vi "Run Multiple Bitfiles.vi"(8 "error in (no error)":errorcluster, 11 "rt data in":T1 {"Compiled Data"."FPGA Data"."1.1 APUs"."shared settings"."cycle start" format="%#.15g"; "Compiled Data"."FPGA Data"."1.0 APUs"."shared settings"."cycle start" format="%#.15g"; "Compiled Data"."1.1 APUs"."shared settings"."cycle start" format="%#.15g"; "Compiled Data"."1.0 APUs"."shared settings"."cycle start" format="%#.15g"}) -> (0 "error out":errorcluster, 3 "rt data out":T1 {"Compiled Data"."FPGA Data"."1.1 APUs"."shared settings"."cycle start" format="%#.15g"; "Compiled Data"."FPGA Data"."1.0 APUs"."shared settings"."cycle start" format="%#.15g"; "Compiled Data"."1.1 APUs"."shared settings"."cycle start" format="%#.15g"; "Compiled Data"."1.0 APUs"."shared settings"."cycle start" format="%#.15g"})   [LabVIEW 2020, in "Engine Simulation Toolkit Engine.lvlib"]
uses:
  Engine Simulation Toolkit Engine.lvlib
  RT Data.ctl
  Shared/Compiled Data.ctl
  Shared/Engine Init Data.ctl
  Shared/1.0 APU Engine Data.ctl
  Shared/1.0 APU Engine FIFO Idxs.ctl
  Shared/Engine Status Data.ctl
  Shared/1.0 Analog Replay Engine Data.ctl
  Shared/1.0 Analog Replay FIFO Idxs.ctl
  Shared/1.0 Digital Pattern Gen Engine Data.ctl
  Shared/1.0 Digital Pattern Gen FIFO Idxs.ctl
  Shared/1.0 Event Timing Capture Engine Data.ctl
  Shared/1.0 Event Timing Capture FIFO Idxs.ctl
  Shared/1.0 Event Timing Measure Engine Data.ctl
  Shared/1.0 Event Timing Measure FIFO Idxs.ctl
  Shared/1.0 Knock Sensor Engine Data.ctl
  Shared/1.0 Knock Sensor FIFO Idxs.ctl
  Shared/1.0 Knock Cylinder Engine Data.ctl
  Shared/1.0 Knock Cylinder FIFO Idxs.ctl
  Shared/1.0 Directional Speed Engine Data.ctl
  Shared/1.0 Directional Speed FIFO Idxs.ctl
  Shared/1.1 APU Engine Data.ctl
  Shared/1.1 Event Timing Measure Engine Data.ctl
  Shared/1.3 Digital Pattern Gen Engine Data.ctl
  Shared/1.3 Digital Pattern Gen FIFO Idxs.ctl
  Shared/Bitfile EST Version.ctl
  Shared/1.3 APU Engine Data.ctl
  Shared/FPGA Datum.ctl
  Shared/1.4 APU Engine Data.ctl
  Shared/1.4 APU Engine FIFO Idxs.ctl
  FPGA Refs.ctl
  APU 1.0 Run Refs.ctl
  APU 1.0 Output Ref.ctl
  APU 1.0 Input Ref.ctl
  Analog Replay 1.0 Input Ref.ctl
  Digital Pattern Gen 1.0 Input Ref.ctl
  Event Timing Capture 1.0 Output Ref.ctl
  Event Timing Measure 1.0 Output Ref.ctl
  Knock Cylinder 1.0 Input Ref.ctl
  Knock Sensor 1.0 Input Ref.ctl
  Directional Speed 1.0 Input Ref.ctl
  Digital Pattern Gen 1.3 Run Refs.ctl
  Digital Pattern Gen 1.3 Settings Ref.ctl
  FPGA Master ref.ctl
  <vilib>/FPGAPlugInAG/Dynamic/niLvFpga_Run_Dynamic.vi
  <vilib>/rvi/interface/nirviMethod/nirviMethod.xnode
  Shared/Engine Simulation Toolkit Shared.lvlib
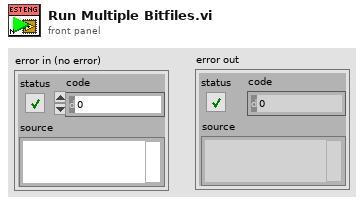
[diagram p1: front panel]
types:
  T1 = typedef "Engine Simulation Toolkit Engine.lvlib/RT Data.ctl" = cluster{"Compiled Data":T2, "FPGA Refs":T30, "FPGA Ref Array":T30[], "Master FPGA ref array":T43[]}
  T2 = typedef "Engine Simulation Toolkit Shared.lvlib/Compiled Data.ctl" = cluster{"Init":T3, "1.0 APUs":T4[], "Status":T6, "DevOutFIFO":refnum<k33>, "DevInFIFO":refnum<k33>, "Device Inputs":dbl[], "Device Outputs":dbl[], "Last Device Inputs":dbl[], "1.0 Analog Replays":T7[], "Unused Analog Replays":string[], "1.0 Digital Pattern Gens":T9[], "Unused Digital Pattern Gens":string[], "1.0 Event Captures":T11[], "1.0 Event Measures":T13[], "1.0 Knock Sensors":T15[], "1.0 Knock Cylinders":T17[], "1.0 Directional Speed":T19[], "Unused Directional Sensors":string[], "1.1 APUs":T21[], "1.1 Event Measures":T22[], "1.3 Digital Pattern Gens":T23[], "Bitfile EST Version":T25, "1.3 APUs":T26[], "Feature Toggles":cluster{"Multi FPGA":bool}, "FPGA Data":T27[]}
  T3 = typedef "Engine Simulation Toolkit Shared.lvlib/Engine Init Data.ctl" = cluster{"CPU":i32, "RIO Address":string, "Decimation":i64, "Priority":i32, "Name":string, "Bitfile Path":path, "Input FIFO Size":i32, "Output FIFO Size":i32, "Master RIO Address":string}
  T4 = typedef "Engine Simulation Toolkit Shared.lvlib/1.0 APU Engine Data.ctl" = cluster{"register names":cluster{"shared settings":string, "input":string, "settings":string, "output":string}, "shared settings":cluster{"cycle start":fxp<+,2,2>, "crank start":u16, "stuck limit":fxp<+,18,18>}, "settings":cluster{"acceleration":fxp<+,18,-20>, "max cycle":fxp<+,2,2>, "enable accel":bool}, "FIFO indexes":T5, "input":cluster{"desired speed":fxp<+/-,23,2>, "reset":bool}, "degrees of 1 cycle u16":dbl, "degrees of 1 crank u16":dbl}
  T5 = typedef "Engine Simulation Toolkit Shared.lvlib/1.0 APU Engine FIFO Idxs.ctl" = cluster{"inputs":cluster{"desired speed":i32, "reset":i32}, "outputs":cluster{"crank angle":i32, "cycle angle":i32, "actual speed":i32}}
  T6 = typedef "Engine Simulation Toolkit Shared.lvlib/Engine Status Data.ctl" = cluster{"FIFO indexes":cluster{"code":i32, "loop duration":i32, "late count":i32}}
  T7 = typedef "Engine Simulation Toolkit Shared.lvlib/1.0 Analog Replay Engine Data.ctl" = cluster{"register names":cluster{"load input":string, "settings":string, "input":string}, "settings":cluster{"ReverseNegate":bool, "CycleAngle":bool, "SpeedThreshold":fxp<+/-,23,2>, "AOBelowThreshold":i16}, "FIFO indexes":T8, "input":cluster{"Offset":i16, "VScaleSlope":fxp<+,18,6>, "VScaleIntercept":fxp<+/-,18,3>}, "offset convert":dbl, "DAC LUT":i16[], "SE_VScaleIntercept":fxp<+/-,18,3>, "SE_VScaleSlope":fxp<+,18,6>, "VOverride":bool, "ResetVolts":bool}
  T8 = typedef "Engine Simulation Toolkit Shared.lvlib/1.0 Analog Replay FIFO Idxs.ctl" = cluster{"enable voltage":i32, "volt slope":i32, "volt intercept":i32, "offset":i32}
  T9 = typedef "Engine Simulation Toolkit Shared.lvlib/1.0 Digital Pattern Gen Engine Data.ctl" = cluster{"register names":cluster{"load input":string, "settings":string, "input":string}, "settings":cluster{"edge 1":u16, "edge 2":u16, "cycle angle":bool, "enabled":bool, "first falling":bool}, "FIFO indexes":T10, "input":cluster{"Offset":i16}, "offset convert":dbl, "Position LUT":u16[]}
  T10 = typedef "Engine Simulation Toolkit Shared.lvlib/1.0 Digital Pattern Gen FIFO Idxs.ctl" = cluster{"offset":i32}
  T11 = typedef "Engine Simulation Toolkit Shared.lvlib/1.0 Event Timing Capture Engine Data.ctl" = cluster{"register names":cluster{"output":string}, "FIFO indexes":T12, "degrees of 1 u16":dbl, "wrap":bool, "window min":u16, "duration convert":dbl, "default start":dbl, "default end":dbl, "ref angle":dbl}
  T12 = typedef "Engine Simulation Toolkit Shared.lvlib/1.0 Event Timing Capture FIFO Idxs.ctl" = cluster{"start angle":i32, "end angle":i32, "duration":i32}
  T13 = typedef "Engine Simulation Toolkit Shared.lvlib/1.0 Event Timing Measure Engine Data.ctl" = cluster{"register names":cluster{"settings":string, "output":string}, "settings":cluster{"max":u16, "min":u16, "active high":bool, "wrap":bool, "full window":bool}, "FIFO indexes":T14}
  T14 = typedef "Engine Simulation Toolkit Shared.lvlib/1.0 Event Timing Measure FIFO Idxs.ctl" = cluster{"stuck active":i32, "win all active":i32, "win orph start":i32, "win orph end":i32}
  T15 = typedef "Engine Simulation Toolkit Shared.lvlib/1.0 Knock Sensor Engine Data.ctl" = cluster{"register names":cluster{"settings":string, "input":string}, "settings":cluster{"low freq (periods/tick)":fxp<+,32,0>, "high freq (periods/tick)":fxp<+,32,0>, "duration (1.25MHz tics)":fxp<+,18,18>, "low freq speed slope":fxp<+,16,-3>, "low freq speed intercept":fxp<+,10,-10>, "low freq by speed":bool}, "DAC multiplier":dbl, "FIFO indexes":T16, "input":cluster{"low freq scaler":fxp<+,10,0>}}
  T16 = typedef "Engine Simulation Toolkit Shared.lvlib/1.0 Knock Sensor FIFO Idxs.ctl" = cluster{"amp":i32}
  T17 = typedef "Engine Simulation Toolkit Shared.lvlib/1.0 Knock Cylinder Engine Data.ctl" = cluster{"register names":cluster{"settings":string, "input":string}, "settings":cluster{"seed":u16, "reset":bool}, "input":cluster{"probability compare":u16, "high freq scaler":fxp<+,10,0>, "trigger position":u16}, "DAC multiplier":dbl, "FIFO indexes":T18, "Angle multiplier":dbl}
  T18 = typedef "Engine Simulation Toolkit Shared.lvlib/1.0 Knock Cylinder FIFO Idxs.ctl" = cluster{"prob":i32, "amp":i32, "pos":i32}
  T19 = typedef "Engine Simulation Toolkit Shared.lvlib/1.0 Directional Speed Engine Data.ctl" = cluster{"register names":cluster{"settings":string, "input":string, "load input":string}, "settings":cluster{"Upper Value":u16, "Lower Value":u16, "Upper Index":fxp<+,10,10>, "Lower Index":fxp<+,10,10>, "Enabled":bool}, "input":cluster{"td (tics)":u16, "tf (tics)":u16, "tr (tics)":u16}, "FIFO indexes":T20, "Tooth Centers LUT":u16[]}
  T20 = typedef "Engine Simulation Toolkit Shared.lvlib/1.0 Directional Speed FIFO Idxs.ctl" = cluster{"td":i32, "tf":i32, "tr":i32}
  T21 = typedef "Engine Simulation Toolkit Shared.lvlib/1.1 APU Engine Data.ctl" = cluster{"register names":cluster{"shared settings":string, "input":string, "settings":string, "output":string, "go":string}, "shared settings":cluster{"cycle start":fxp<+,2,2>, "crank start":u16, "stuck limit":fxp<+,18,18>}, "settings":cluster{"acceleration":fxp<+,18,-20>, "max cycle":fxp<+,2,2>, "enable accel":bool}, "FIFO indexes":T5, "input":cluster{"desired speed":fxp<+/-,23,2>, "reset":bool}, "degrees of 1 cycle u16":dbl, "degrees of 1 crank u16":dbl}
  T22 = typedef "Engine Simulation Toolkit Shared.lvlib/1.1 Event Timing Measure Engine Data.ctl" = cluster{"register names":cluster{"settings":string, "output":string}, "settings":cluster{"max":u16, "min":u16, "active high":bool, "wrap":bool}, "FIFO indexes":T14}
  T23 = typedef "Engine Simulation Toolkit Shared.lvlib/1.3 Digital Pattern Gen Engine Data.ctl" = cluster{"register names":cluster{"load input":string, "settings":string, "input":string}, "settings":cluster{"edge 1":u16, "edge 2":u16, "cycle angle":bool, "enabled":bool, "first falling":bool, "fault":bool, "fault wrap":bool, "fault value":bool, "fault count":fxp<+,4,4>, "use fault count":bool}, "FIFO indexes":T24, "input":cluster{"Offset":i16}, "deg to u16 scale":dbl, "Position LUT":u16[], "# of teeth":i16, "max angle":dbl}
  T24 = typedef "Engine Simulation Toolkit Shared.lvlib/1.3 Digital Pattern Gen FIFO Idxs.ctl" = cluster{"offset":i32, "command":i32, "rotations":i32, "start angle":i32, "stop angle":i32, "tooth to rem":i32, "trigger":i32, "valid":i32}
  T25 = typedef "Engine Simulation Toolkit Shared.lvlib/Bitfile EST Version.ctl" = enum16{"1.0", "1.1", "1.2", "1.3", "1.4"}
  T26 = typedef "Engine Simulation Toolkit Shared.lvlib/1.3 APU Engine Data.ctl" = cluster{"register names":cluster{"shared settings":string, "input":string, "settings":string, "output":string, "go":string}, "shared settings":cluster{"start":fxp<+,17,17>, "stuck limit":fxp<+,18,18>}, "settings":cluster{"acceleration":fxp<+,18,-20>, "enable accel":bool}, "FIFO indexes":T5, "input":cluster{"desired speed":fxp<+/-,23,2>, "reset":bool}, "degrees of 1 cycle u16":dbl, "degrees of 1 crank u16":dbl}
  T27 = typedef "Engine Simulation Toolkit Shared.lvlib/FPGA Datum.ctl" = cluster{"Bitfile Path":path, "RIO Address":string, "1.0 APUs":T4[], "Unused Analog Replays":string[], "1.0 Digital Pattern Gens":T9[], "Unused Digital Pattern Gens":string[], "1.0 Event Captures":T11[], "Unused Directional Sensors":string[], "1.1 APUs":T21[], "1.0 Directional Speed":T19[], "1.0 Analog Replays":T7[], "1.0 Event Measures":T13[], "1.0 Knock Sensors":T15[], "1.0 Knock Cylinders":T17[], "1.1 Event Measures":T22[], "1.3 Digital Pattern Gens":T23[], "Bitfile EST Version":T25, "1.3 APUs":T26[], "1.4 APUs":T28[]}
  T28 = typedef "Engine Simulation Toolkit Shared.lvlib/1.4 APU Engine Data.ctl" = cluster{"register names":cluster{"shared settings":string, "input":string, "settings":string, "output":string, "go":string, "master":string, "send trigger":string}, "shared settings":cluster{"start":fxp<+,17,17>, "stuck limit":fxp<+,18,18>}, "settings":cluster{"acceleration":fxp<+,18,-20>, "enable accel":bool}, "FIFO indexes":T29, "input":cluster{"desired speed":fxp<+/-,23,2>, "reset":bool}, "degrees of 1 cycle u16":dbl, "degrees of 1 crank u16":dbl, "max deviation angle":dbl}
  T29 = typedef "Engine Simulation Toolkit Shared.lvlib/1.4 APU Engine FIFO Idxs.ctl" = cluster{"inputs":cluster{"desired speed":i32, "reset":i32}, "outputs":cluster{"crank angle":i32, "cycle angle":i32, "actual speed":i32, "devices synchronized":i32, "deviation error":i32}}
  T30 = typedef "Engine Simulation Toolkit Engine.lvlib/FPGA Refs.ctl" = cluster{"1.0 APUs":T31[], "FPGA ref":refnum<k20>, "1.0 Analog Replays":T34[], "1.0 Dig Pat Gens":T35[], "1.0 Event Captures":T36[], "1.0 Event Measures":T37[], "1.0 Knock Cylinders":T38[], "1.0 Knock Sensors":T39[], "1.0 Directional Speed Sensors":T40[], "1.3 Dig Pat Gens":T41[]}
  T31 = typedef "Engine Simulation Toolkit Engine.lvlib/APU 1.0 Run Refs.ctl" = cluster{"output reference":T32, "input reference":T33}
  T32 = typedef "Engine Simulation Toolkit Engine.lvlib/APU 1.0 Output Ref.ctl" = refnum<k20>
  T33 = typedef "Engine Simulation Toolkit Engine.lvlib/APU 1.0 Input Ref.ctl" = refnum<k20>
  T34 = typedef "Engine Simulation Toolkit Engine.lvlib/Analog Replay 1.0 Input Ref.ctl" = refnum<k20>
  T35 = typedef "Engine Simulation Toolkit Engine.lvlib/Digital Pattern Gen 1.0 Input Ref.ctl" = refnum<k20>
  T36 = typedef "Engine Simulation Toolkit Engine.lvlib/Event Timing Capture 1.0 Output Ref.ctl" = refnum<k20>
  T37 = typedef "Engine Simulation Toolkit Engine.lvlib/Event Timing Measure 1.0 Output Ref.ctl" = refnum<k20>
  T38 = typedef "Engine Simulation Toolkit Engine.lvlib/Knock Cylinder 1.0 Input Ref.ctl" = refnum<k20>
  T39 = typedef "Engine Simulation Toolkit Engine.lvlib/Knock Sensor 1.0 Input Ref.ctl" = refnum<k20>
  T40 = typedef "Engine Simulation Toolkit Engine.lvlib/Directional Speed 1.0 Input Ref.ctl" = refnum<k20>
  T41 = typedef "Engine Simulation Toolkit Engine.lvlib/Digital Pattern Gen 1.3 Run Refs.ctl" = cluster{"input":T35, "settings":T42}
  T42 = typedef "Engine Simulation Toolkit Engine.lvlib/Digital Pattern Gen 1.3 Settings Ref.ctl" = refnum<k20>
  T43 = typedef "Engine Simulation Toolkit Engine.lvlib/FPGA Master ref.ctl" = cluster{"Master ctl ref":refnum<k20>, "Send Trigger ref":refnum<k20>}
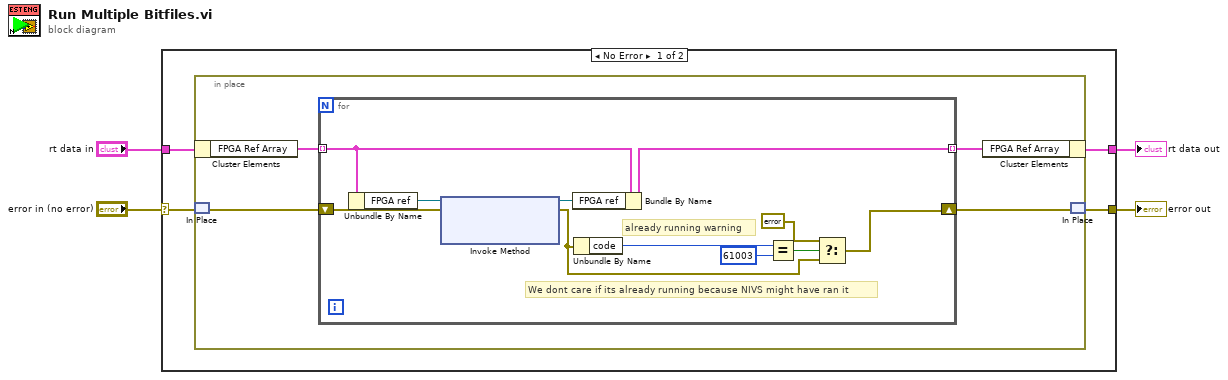
[diagram p0: block diagram]
diagram:
  n1 = case shown="No Error" "error in (no error)" {
    selector: "error in (no error)" -> [w6 w24]
    tunnel: "rt data in" -> [w8 w25]
    tunnel: [w7 w25] -> w1
    tunnel: [w5 w24] -> w2
    frame No Error {
      n2 = in-place {
        n3 = in-place-cluster #1(w8) -> ("FPGA Ref Array"=w12:T30[])
        n4 = in-place-match #2(w6) -> (w10:errorcluster)
        n5 = for {
          shift-right: [w19] -> w9
          shift-left: w10 -> [w18]
          tunnel: w12 -> [w15] mode=indexing
          tunnel: [w13] -> w11 mode=indexing
          # "We dont care if its already running because NIVS might have ran it"
          # "already running warning"
          n6 = Unbundle By Name(w15) -> ("FPGA ref"=w16:refnum<k20>)
          n7 = xnode "Invoke Method"("FPGA VI Reference In"=w16, "error in"=w18) -> ("FPGA VI Reference Out"=w14:refnum<k20>, "error out"=w17:errorcluster)  [unwired: 1 in]
          n8 = Bundle By Name(cluster=w15, "FPGA ref"=w14) -> (w13:T30)
          n9 = Unbundle By Name(w17) -> ("code"=w23:i32)
          n10 = Equal?(x=w23, y=61003) -> (x = y?=w21:bool)
          n11 = Select(t=errorcluster {"status"=FALSE, "code"=0, "source"=""}, s=w21, f=w17) -> (s? t:f=w19:errorcluster)
        }
        n12 = in-place-cluster #1("FPGA Ref Array"=w11) -> (w7:T1)
        n13 = in-place-match #2(w9) -> (w5:errorcluster)
      }
    }
    frame Error {
    }
  }
  "error out" <- w2
  "rt data out" <- w1
